vi "Output Data.vi"() -> ()   [LabVIEW 2013]
uses:
  qwtb_lvlib/TD Quantity.ctl
  globals.vi
panel:
  in  "new data signal":bool
  in  "close":bool
  out "Selected Quantity":T1={"Name"="", "Value"=[[1.0]], "Uncertainty"=[[1.0]], "Degrees of\nFreedom"=[[10.0]], "Correlation"=[[10.0]], "Randomized uncertainty"=[[10.0]]}
  in  "Q list":i32(listbox) caption="Input Quantities"
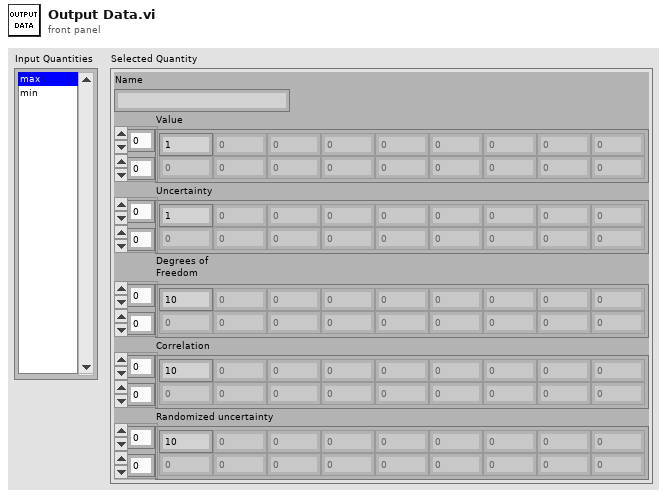
[diagram p1: front panel]
types:
  T1 = typedef "TD Quantity.ctl" = cluster{"Name":string, "Value":dbl[][], "Uncertainty":dbl[][], "Degrees of\nFreedom":dbl[][], "Correlation":dbl[][], "Randomized uncertainty":dbl[][]}
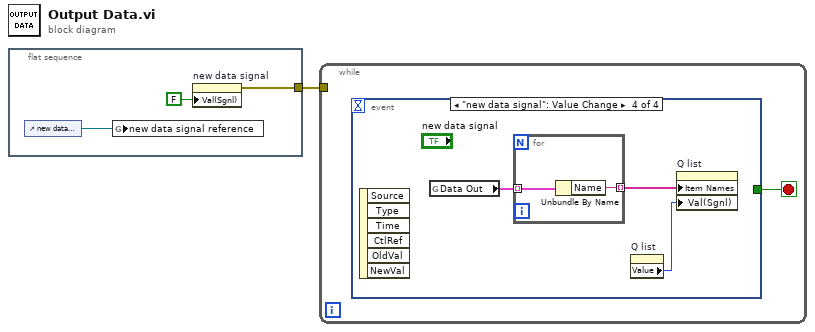
[diagram p0: block diagram]
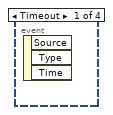
[diagram p2: hidden frame]
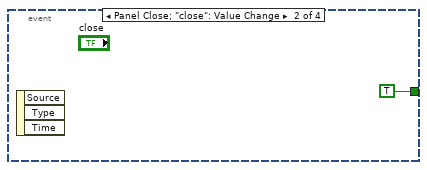
[diagram p3: hidden frame]
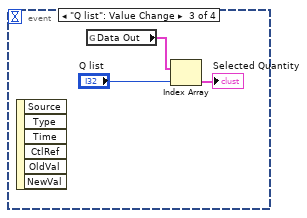
[diagram p4: hidden frame]
diagram:
  n1 = flat-sequence {
    tunnel: [w2] -> w1
    frame #0 {
      n2 = control-ref of="new data signal"() -> (w4:refnum<vi>)
      n3 = global write "globals.vi" "new data signal reference"(w4) -> ()
      n4 = property on="new data signal" class="Bool (strict)"("Val(Sgnl)"=FALSE ("Value (Signaling)")) -> (error out=w2:errorcluster)  [unwired: 2 in, 1 out]
    }
  }
  n5 = while {
    tunnel: w1 -> [_]
    stop <- w5 stop-if-true
    n6 = event shown="[3] \"new data signal\": Value Change" {
      selector: _ -> [_ _ _ _]
      dyn-events: _ -> [_ _ _ _]
      timeout: _ -> [_ _ _ _]
      tunnel: [_ TRUE _ _] -> w5
      event Timeout {
        n7 = event-data() -> ()  [unwired: 1 in, 3 out]
      }
      event Panel Close; "close": Value Change {
        n8 = event-data() -> ()  [unwired: 1 in, 3 out]
      }
      event "Q list": Value Change {
        n9 = event-data() -> ()  [unwired: 1 in, 6 out]
        n10 = global read "globals.vi" "Data Out"() -> (w9:T1[])
        n11 = Index Array(array=w9, index="Q list") -> (element=→"Selected Quantity":T1)
      }
      event "new data signal": Value Change {
        n12 = event-data() -> ()  [unwired: 1 in, 6 out]
        n13 = global read "globals.vi" "Data Out"() -> (w12:T1[])
        n14 = for {
          tunnel: [w14] -> w11 mode=indexing
          tunnel: w12 -> [w13] mode=indexing
          n15 = Unbundle By Name(w13) -> ("Name"=w14:string)
        }
        n16 = property on="Q list" class="LstBox (strict)"() -> ("Value"=w10:i32)  [unwired: 2 in, 2 out]
        n17 = property on="Q list" class="LstBox (strict)"("Item Names"=w11, "Val(Sgnl)"=w10) -> ()  [unwired: 2 in, 2 out]
      }
    }
  }
